vi "open configuration.vi"(4 "error in":errorcluster, 6 "file path":path) -> (0 "error out":errorcluster, 3 "Channel Indices":T1[](array[typedef]))   [LabVIEW 2015]
uses:
  DAQ configuration/channel identifier.ctl
  file action.ctl
  DAQ configuration/Sensor buffer command.ctl
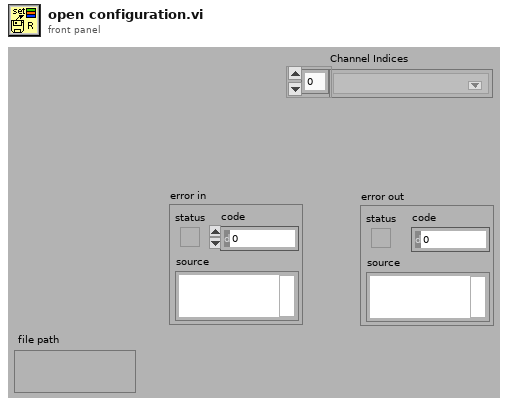
[diagram p1: front panel]
types:
  T1 = typedef "channel identifier.ctl" = u16
  T2 = typedef "Sensor buffer command.ctl" = enum16{"read average", "read recent", "read all", "write", "set buffer size", "Read channel config", "Write channel config", "clear"}
  T3 = typedef "file action.ctl" = enum16{"Save", "Open"}
  T4 = typedef "Channel config.ctl" = cluster{"Channel Indices":T1[], "AI Max voltage":dbl[], "Calibration matrix":T5}
  T5 = typedef "calib array.ctl" = T6[]
  T6 = typedef "conversion.ctl" = cluster{"conversion matrix":sgl[][], "units":string, "name":string, "scale type":T7, "offset (volts)":dbl, "second channel":i8, "correspondence table":T8, "offset (physical units)":dbl, "pH scale":T9, "D.O.":T10, "Photometer data":T11}
  T7 = typedef "scale type.ctl" = enum16{"Volts", "Polynomial", "Correspondence Table", "pH", "Dissolved Oxygen", "Quadratic", "Photometer"}
  T8 = typedef "correspondence table.ctl" = cluster{"physical units":dbl, "volts":dbl}[]
  T9 = typedef "pH scale.ctl" = cluster{"Buffers":cluster{"Buffer":dbl, "Calibrated":bool, "V/T":dbl}[], "Temperature":dbl}
  T10 = typedef "DO scale.ctl" = cluster{"Temperature":dbl, "K":dbl, "barometric pressure":dbl}
  T11 = typedef "Photometer calibration data.ctl" = cluster{"Dark Voltage":dbl, "Blank Voltage":dbl, "Standards":cluster{"Concentration":dbl, "Voltage":dbl}[]}
  T12 = cluster{"Channel Indices":T1[], "Calibration matrix":T5}
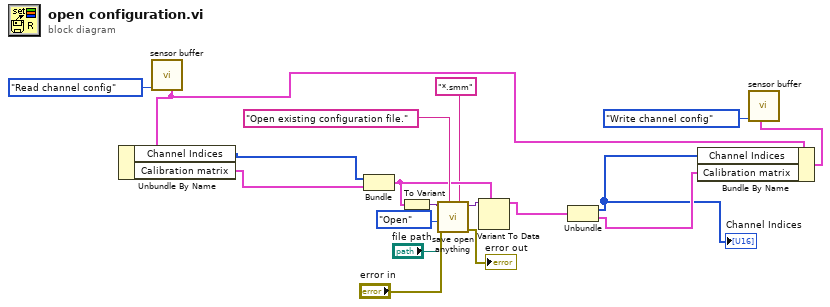
[diagram p0: block diagram]
diagram:
  n1 = call "sensor buffer.vi"("command"=Sensor_buffer_command."Read channel config") -> ("Channel Config out"=w4:T4)  [unwired: 6 in, 4 out]
  n2 = Unbundle By Name(w4) -> ("Channel Indices"=w7:T1[], "Calibration matrix"=w6:T5)
  n3 = Bundle("Channel Indices"=w7, "Calibration matrix"=w6) -> (w14:T12)  [unwired: 1 in]
  n4 = To Variant(anything=w14) -> (Variant=w17:variant)
  n5 = call "save open anything.vi"("Variant"=w17, "file path"="file path", "Action"=file_action."Open", "error in (not an error)"="error in", "prompt"="Open existing configuration file.", "pattern"="*.smm") -> ("Variant out"=w18:variant, "error out"=→"error out":errorcluster)  [unwired: 1 in, 2 out]
  n6 = Variant To Data(type=w14, Variant=w18) -> (data=w13:T12)  [unwired: 1 in, 1 out]
  n7 = Unbundle(w13) -> ("Channel Indices"=w1:T1[], "Calibration matrix"=w3:T5)
  "Channel Indices" <- w1
  n8 = Bundle By Name(cluster=w4, "Channel Indices"=w1, "Calibration matrix"=w3) -> (w2:T4)
  n9 = call "sensor buffer.vi"("Channel Config"=w2, "command"=Sensor_buffer_command."Write channel config") -> ()  [unwired: 5 in, 5 out]
